vi "dfd_Check Waveform Fs Consistency.vi"(7 "init in":bool, 8 "error in (no error)":errorcluster, 9 "signal in":waveform(dbl), 10 "dt in":dbl) -> (0 "error out":errorcluster, 1 "signal out":waveform(dbl), 2 "dt out":dbl, 5 "init out":bool)   [LabVIEW 2017, in "NI_DigFilter_Process.lvlib"]
uses:
  <vilib>/addons/Digital Filter Design/NI_DigFilter_Process.lvlib
  <vilib>/addons/Digital Filter Design/_Misc.llb/dfd_Error Handlers (Single).vi
  <vilib>/addons/Digital Filter Design/NI_DigFilterLicensed.lvlib
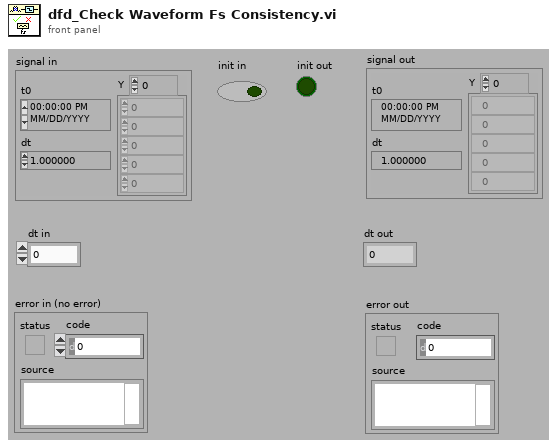
[diagram p1: front panel]
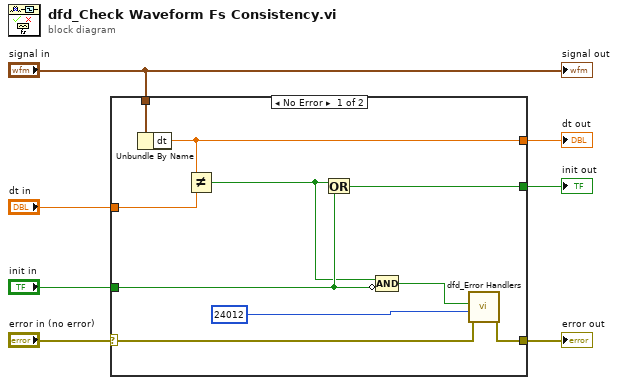
[diagram p0: block diagram]
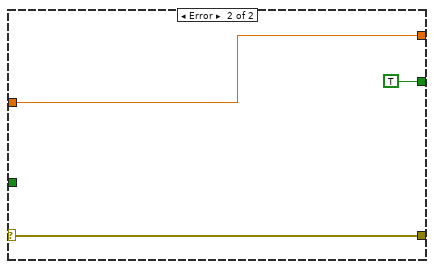
[diagram p2: hidden frame]
diagram:
  n1 = case shown="No Error" "error in (no error)" {
    selector: "error in (no error)" -> [w10 w20]
    tunnel: "signal in" -> [w17 _]
    tunnel: [w16 TRUE] -> w7
    tunnel: "init in" -> [w15 _]
    tunnel: [w11 w20] -> w5
    tunnel: "dt in" -> [w9 w19]
    tunnel: [w8 w19] -> w1
    frame No Error {
      n2 = Unbundle By Name(w17) -> ("dt"=w8:dbl)
      n3 = Not Equal?(x=w8, y=w9) -> (x != y?=w14:bool)
      n4 = Or(x=w14, y=w15) -> (x .or. y?=w16:bool)
      n5 = Compound Arithmetic op=AND(w14, invert w15) -> (w13:bool)
      n6 = call-poly <vilib>:"dfd_Error Handlers.vi"("error in (no error)"=w10, "error code"=24012 ("WRN_PROC_FS_INCONSISTENT"), "condition failed?"=w13) -> ("error out"=w11:errorcluster)  [unwired: 8 out]
    }
    frame Error {
    }
  }
  "error out" <- w5
  "init out" <- w7
  "dt out" <- w1
  "signal out" <- "signal in"
